vi "AllCosWindow (CDB).vi"(4 "scale?":bool, 5 "window":u16(ring) items=["None "=0, "Hanning"=1, "Hamming"=2, "Blackman-Harris"=3, "Exact Blackman"=4, "Blackman"=5, "Flat Top"=6, "4 Term B-Harris "=7, "7 Term B-Harris"=8, "Low Sidelobe"=9, "Blackman Nuttall"=11], 6 "X":cdb[](array[numeric])) -> (0 "error":i32, 2 "Windowed X":cdb[](array[numeric]))   [LabVIEW 2022 SP3, in "NI_AALPro.lvlib"]
uses:
  NI_AALPro.lvlib
  <resource>/lvanlys.dll
panel:
  # "Cosine Window"
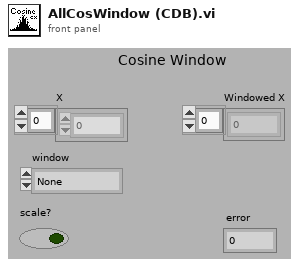
[diagram p1: front panel]
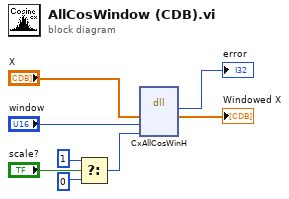
[diagram p0: block diagram]
diagram:
  n1 = Select(t=1, s="scale?", f=0) -> (s? t:f=w1:i32)
  n2 = dll-call lib="C:/Program Files (x86)/National Instruments/LabVIEW 2022/resource/lvanlys.*" fn="CxAllCosWinH"("X"="X", "winType"="window", "scaled"=w1) -> (→"error":i32, "X"=→"Windowed X":cdb[])  [unwired: 4 in, 3 out]
